vi "pf_Get_Property_Info_from_index.vi"(8 "error in (no error)":errorcluster, 10 "Property index":i32, 11 "IMAQ Session in":refnum<k11>) -> (0 "error out":errorcluster, 1 "Property Flag":i32, 2 "Property Type":i32, 3 "IMAQ Session out":refnum<k11>, 5 "Property Name":string)   [LabVIEW 2025, in "Photonfocus_Toolkit.lvlib"]
uses:
  Photonfocus_Toolkit.lvlib
  _Private/Controls/pf_Camera_ctrl_mngr_action.ctl
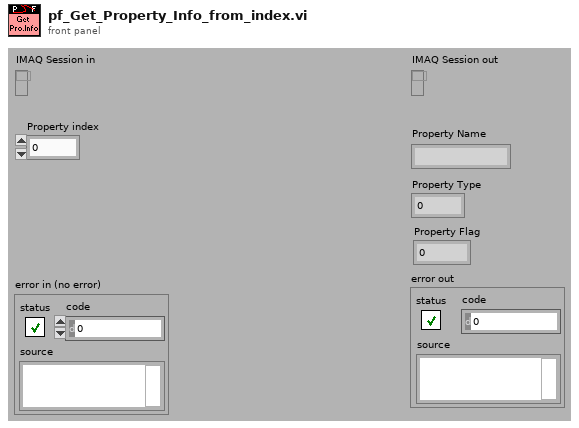
[diagram p1: front panel]
types:
  T1 = typedef "Photonfocus_Toolkit.lvlib/pf_Camera_ctrl_mngr_action.ctl" = enum16{"Create", "Destroy", "Set", "Get"}
  T2 = typedef "Photonfocus_Toolkit.lvlib/pf_Camera_Control.ctl" = cluster{"Port Name":string, "Port Number":i32, "IMAQ Session":refnum<k11>, "PeakDetector_Mode":T3, "Window.W":u32, "Window.H":u32}
  T3 = typedef "Photonfocus_Toolkit.lvlib/pf_PeakDetector_Mode.ctl" = enum16{"Undefined", "2D only", "2D and 3D", "3D only"}
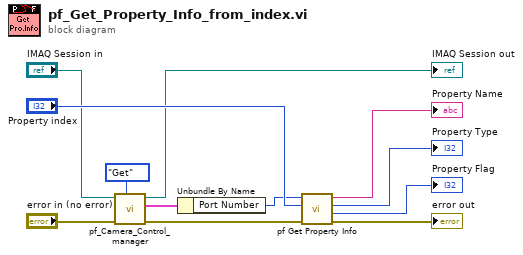
[diagram p0: block diagram]
diagram:
  n1 = call "pf_Camera_Control_manager.vi"("Action"=pf_Camera_ctrl_mngr_action."Get", "error in (no error)"="error in (no error)", "IMAQ Session in"="IMAQ Session in") -> ("error out"=w6:errorcluster, "Camera Control out"=w4:T2, "IMAQ Session out"=→"IMAQ Session out":refnum<k11>)  [unwired: 1 in, 5 out]
  n2 = Unbundle By Name(w4) -> ("Port Number"=w3:i32)
  n3 = call "pf Get Property Info.vi"("error in (no error)"=w6, "iProperty"="Property index", "iPort"=w3) -> ("error out"=→"error out":errorcluster, "iPropFlag"=→"Property Flag":i32, "iPropType"=→"Property Type":i32, "function return"=→"Property Name":string)  [unwired: 5 out]
